vi "Error Query.vi"(8 "error in (no error)":errorcluster, 11 "VISA resource name":refnum<visa-resource-name>) -> (0 "error out":errorcluster, 1 "Error Message":string, 2 "Error Code":i32[](array[numeric]), 3 "VISA resource name out":refnum<visa-resource-name>)   [LabVIEW 2025]
doc: "Queries the instrument for any errors in the instrument's error queue. It will continue to read errors until all errors have been read from the instrument. Any errors will be returned in the <B>error out</B> control.\n\n<B>Note:</B>\nThis VI is called automatically by most driver VIs so it is not usually necessary to call this in an application."
panel:
  # "EDIT: Note: The Error Query VI is included as a subVI in all driver VIs except low-level API VIs. If the instrument does not support error query, then remove the VI and remove subVI calls in each instrument driver VI that calls it."
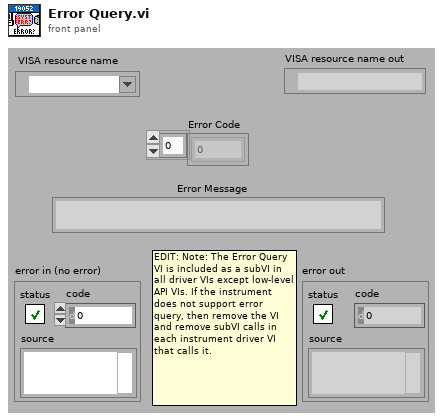
[diagram p1: front panel]
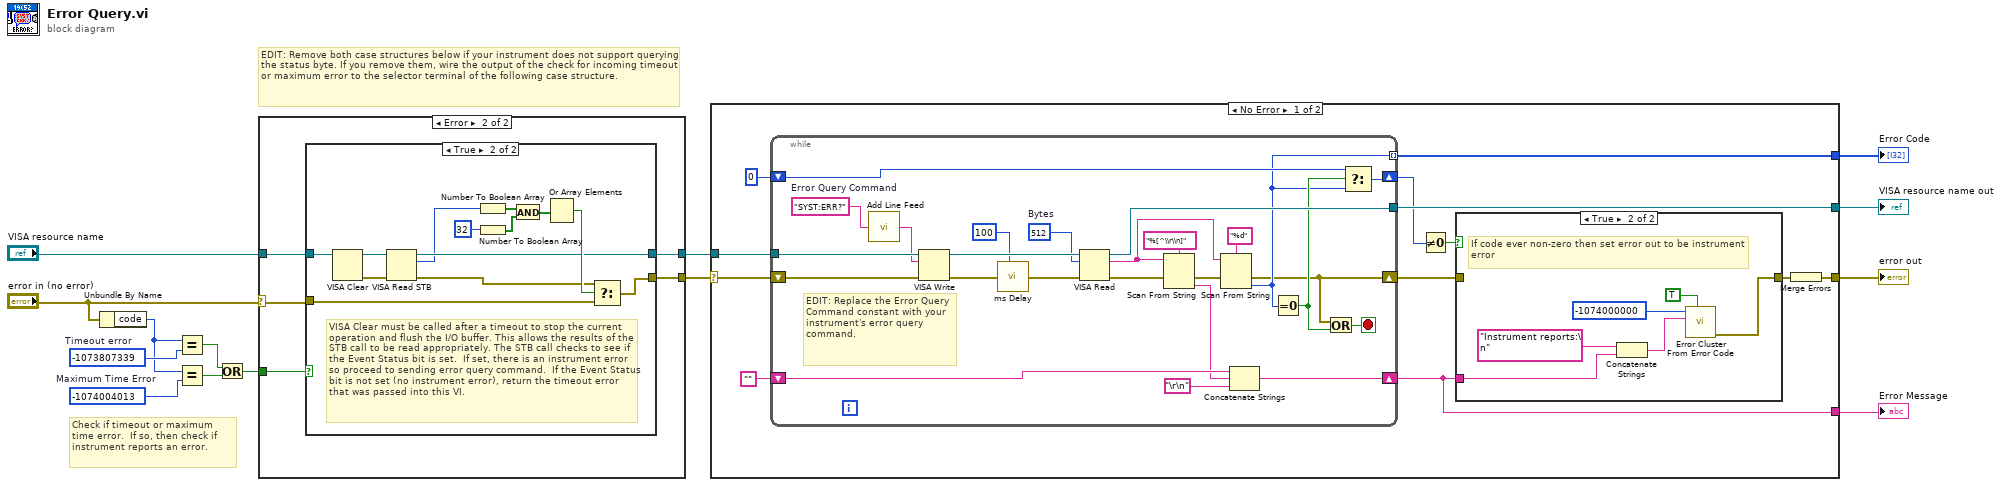
[diagram p0: block diagram]
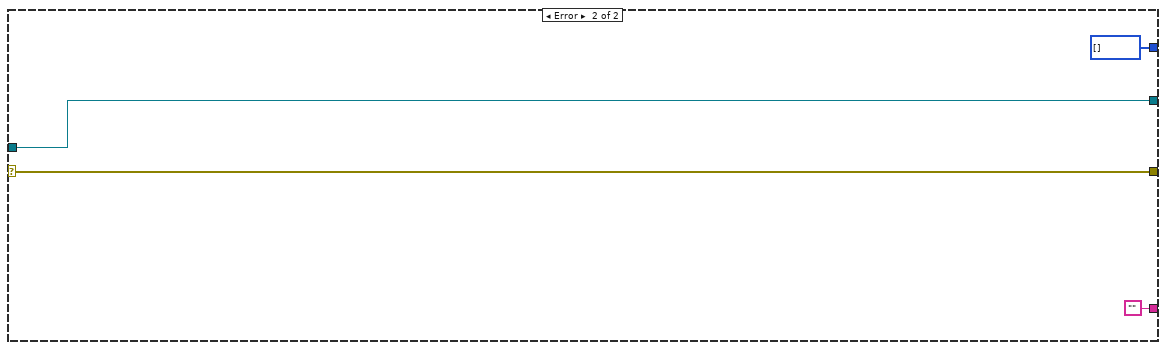
[diagram p5: hidden frame]
diagram:
  w11 = -1074004013  # Maximum Time Error
  w13 = -1073807339  # Timeout error
  # "EDIT: Remove both case structures below if your instrument does not support querying the status byte. If you remove them, wire the output of the check for incoming timeout or maximum error to the selector terminal of the following case structure."
  # "Check if timeout or maximum time error.  If so, then check if instrument reports an error."
  n1 = Unbundle By Name("error in (no error)") -> ("code"=w12:i32)
  n2 = Equal?(x=w12, y=w13) -> (x = y?=w9:bool)
  n3 = Equal?(x=w12, y=w11) -> (x = y?=w10:bool)
  n4 = Or(x=w9, y=w10) -> (x .or. y?=w8:bool)
  n5 = case shown="Error" "error in (no error)" {
    selector: "error in (no error)" -> [w15 w19]
    tunnel: "VISA resource name" -> [w16 w21]
    tunnel: [w16 w20] -> w1
    tunnel: [w15 w18] -> w14
    tunnel: w8 -> [_ w17]
    frame No Error {
    }
    frame Error {
      n6 = case shown="True" w17 {
        tunnel: w21 -> [w23 w29]
        tunnel: [w23 w26] -> w20
        tunnel: w19 -> [w22 w32]
        tunnel: [w22 w31] -> w18
        frame False {
          # "Error code not a timeout, so best to pass on to user."
        }
        frame True {
          # "VISA Clear must be called after a timeout to stop the current operation and flush the I/O buffer. This allows the results of the  STB call to be read appropriately. The STB call checks to see if the Event Status bit is set.  If set, there is an instrument error so proceed to sending error query command.  If the Event Status bit is not set (no instrument error), return the timeout error that was passed into this VI."
          n7 = VISA Clear(VISA resource name=w29) -> (VISA resource name out=w28:refnum<visa-resource-name>, error out=w27:errorcluster)  [unwired: 1 in]
          n8 = VISA Read STB(8:w27, 11:w28) -> (0:w25:errorcluster, 2:w24:u16, 3:w26:refnum<visa-resource-name>)
          n9 = Number To Boolean Array(number=w24) -> (Boolean array=w33:bool[])
          n10 = Number To Boolean Array(number=32) -> (Boolean array=w35:bool[])
          n11 = And(x=w33, y=w35) -> (x .and. y?=w34:bool[])
          n12 = Or Array Elements(Boolean array=w34) -> (logical OR=w30:bool)
          n13 = Select(t=w25, s=w30, f=w32) -> (s? t:f=w31:errorcluster)
        }
      }
    }
  }
  n14 = case shown="No Error" w14 {
    selector: w14 -> [w37 w81]
    tunnel: [w48 w84] -> w3
    tunnel: w1 -> [w47 w84]
    tunnel: [w45 w81] -> w4
    tunnel: [w40 ""] -> w5
    tunnel: [w39 i32[] []] -> w2
    frame No Error {
      n15 = while {
        tunnel: [w79] -> w48
        tunnel: w47 -> [w78]
        shift-right: [w70] -> w40
        shift-left: "" -> [w73]
        shift-right: [w68] -> w41
        shift-left: 0 -> [w69]
        shift-right: [w62] -> w38
        shift-left: w37 -> [w67]
        tunnel: [w63] -> w39 mode=indexing
        stop <- w76 stop-if-true
        w61 = u32 512  # Bytes
        w57 = "SYST:ERR?"  # Error Query Command
        # "EDIT: Replace the Error Query Command constant with your instrument's error query command."
        n16 = call "Add Line Feed.vi"("Command string"=w57) -> ("Concatenated string"=w56:string)  [unwired: 4 in]
        n17 = VISA Write(VISA resource name=w78, write buffer=w56, error in (no error)=w67) -> (VISA resource name out=w80:refnum<visa-resource-name>, error out=w60:errorcluster)  [unwired: 1 out]
        n18 = call "ms Delay.vi"("miliseconds to wait"=u32 100 ("milliseconds to wait"), "error in (no error)"=w60) -> ("error out"=w59:errorcluster)  [unwired: 6 in, 1 out]
        n19 = VISA Read(VISA resource name=w80, byte count=w61, error in (no error)=w59) -> (VISA resource name out=w79:refnum<visa-resource-name>, read buffer=w74:string, error out=w66:errorcluster)  [unwired: 1 out]
        n20 = Scan From String(format string="%[^\\r\\n]", input string=w74, error in=w66) -> (error out=w65:errorcluster, output 1=w71:string)  [unwired: 2 in, 2 out]
        n21 = Scan From String(format string="%d", input string=w74, error in=w65) -> (error out=w62:errorcluster, output 1=w63:i32)  [unwired: 2 in, 2 out]
        n22 = Concatenate Strings(w73, w71, "\r\n") -> (w70:string)
        n23 = Equal To 0?(x=w63) -> (x = 0?=w64:bool)
        n24 = Or(x=w62, y=w64) -> (x .or. y?=w76:bool)
        n25 = Select(t=w69, s=w64, f=w63) -> (s? t:f=w68:i32)
      }
      n26 = Not Equal To 0?(x=w41) -> (x != 0?=w43:bool)
      n27 = case shown="True" w43 {
        tunnel: w40 -> [_ w54]
        tunnel: [w49 w50] -> w42
        tunnel: w38 -> [w49 _]
        frame False {
        }
        frame True {
          # "If code ever non-zero then set error out to be instrument error"
          n28 = Concatenate Strings("Instrument reports:\n" ("Source"), w54) -> (w51:string)
          n29 = call <vilib>:"Error Cluster From Error Code.vi"("show call chain? (False)"=TRUE, "error message (\"\")"=w51, "error code (0)"=-1074000000 ("Code")) -> ("error out"=w50:errorcluster)  [unwired: 6 in]
        }
      }
      n30 = Merge Errors(w42) -> (w45:errorcluster)
    }
    frame Error {
    }
  }
  "VISA resource name out" <- w3
  "error out" <- w4
  "Error Message" <- w5
  "Error Code" <- w2
